vi "RemoveFreeField.vi"(8 "error in (no error)":errorcluster, 10 "Coordinate":cluster{"x":i16, "y":i16}, 11 "SnakeGame in":refnum<class "SnakeGame.lvclass">) -> (0 "error out":errorcluster, 3 "SnakeGame out":refnum<class "SnakeGame.lvclass">)   [LabVIEW 2019, in "RT_Game.lvlib" / "SnakeGame.lvclass"]
uses:
  SnakeGame.lvclass
  SnakeGame.lvclass/SnakeGame.ctl
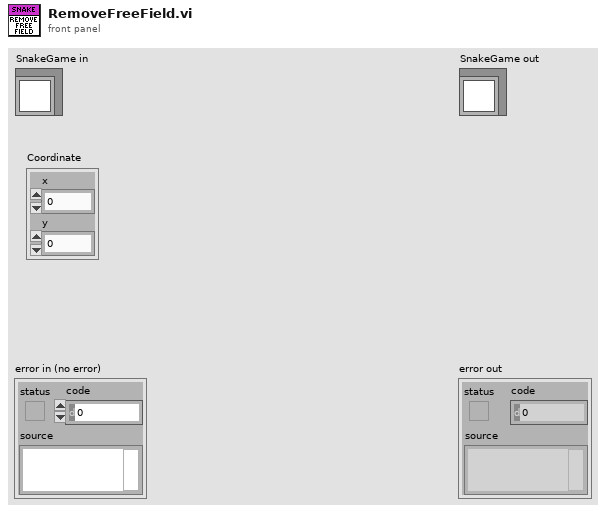
[diagram p1: front panel]
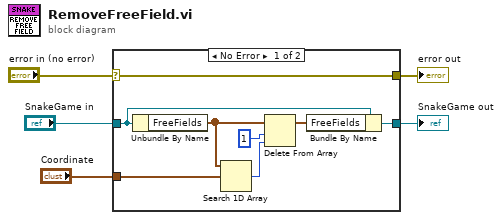
[diagram p0: block diagram]
diagram:
  n1 = case shown="No Error" "error in (no error)" {
    selector: "error in (no error)" -> [w13 w15]
    tunnel: [w13 w15] -> w4
    tunnel: [w12 w14] -> w2
    tunnel: "SnakeGame in" -> [w11 w14]
    tunnel: "Coordinate" -> [w9 _]
    frame No Error {
      n2 = Unbundle By Name(w11) -> ("FreeFields"=w10:cluster{"x":i16, "y":i16}[])
      n3 = Search 1D Array(1D array=w10, element=w9) -> (index of element=w7:i32)  [unwired: 1 in]
      n4 = Delete From Array(array=w10, length=1, index=w7) -> (array with subset deleted=w8:cluster{"x":i16, "y":i16}[])  [unwired: 1 out]
      n5 = Bundle By Name(cluster=w11, "FreeFields"=w8) -> (w12:refnum<class "SnakeGame.lvclass">)
    }
    frame Error {
    }
  }
  "error out" <- w4
  "SnakeGame out" <- w2
